vi "ContourPlot v3.6-IV.vi"() -> ()   [LabVIEW 2019]
uses:
  diff para.ctl
  graph para.ctl
panel:
  out "smoothed dIV buffer":dbl[][](array[numeric])
  in  "diff para":T1={"x0"=-1.0, "Ic0"=2.0, "h0"=1.0, "y0"=0.0}
  in  "Plot reference":bool caption="load data"
  out "smoothed dIV":dbl[][](array[numeric])
  out "smoothed data":dbl[][](array[numeric])
  in  "smooth n":i32=10
  out "IVdata":dbl[][](array[numeric])
  in  "load data":bool
  out "Status":string
  in  "stop":bool
  in  "Begin":i32=1000
  in  "length":i32=1000
  in  "Contact Resistance":dbl
  in  "Tab Control 2":enum32{"IV plots", "IV smoothed", "dV/dI"}(tab)
  out "IV Intensity":dbl[][](graph)
  out "IV":cluster{dbl[], "Intensity Graph":dbl[]}(graph)
  in  "Plot contour line":bool
  out "IV smoothed intensity":dbl[][](graph)
  out "Smooth IV":cluster{dbl[], "Intensity Graph":dbl[]}(graph)
  out "dVdI Intensity":dbl[][](graph)
  out "dV/dI":cluster{dbl[], "Intensity Graph":dbl[]}(graph)
  in  "book number":i32=414
  in  "file path (dialog if empty)":path=path "C:/Users/gyue/Box/Guang Yue uiuc research box folder/data/Contour plot"
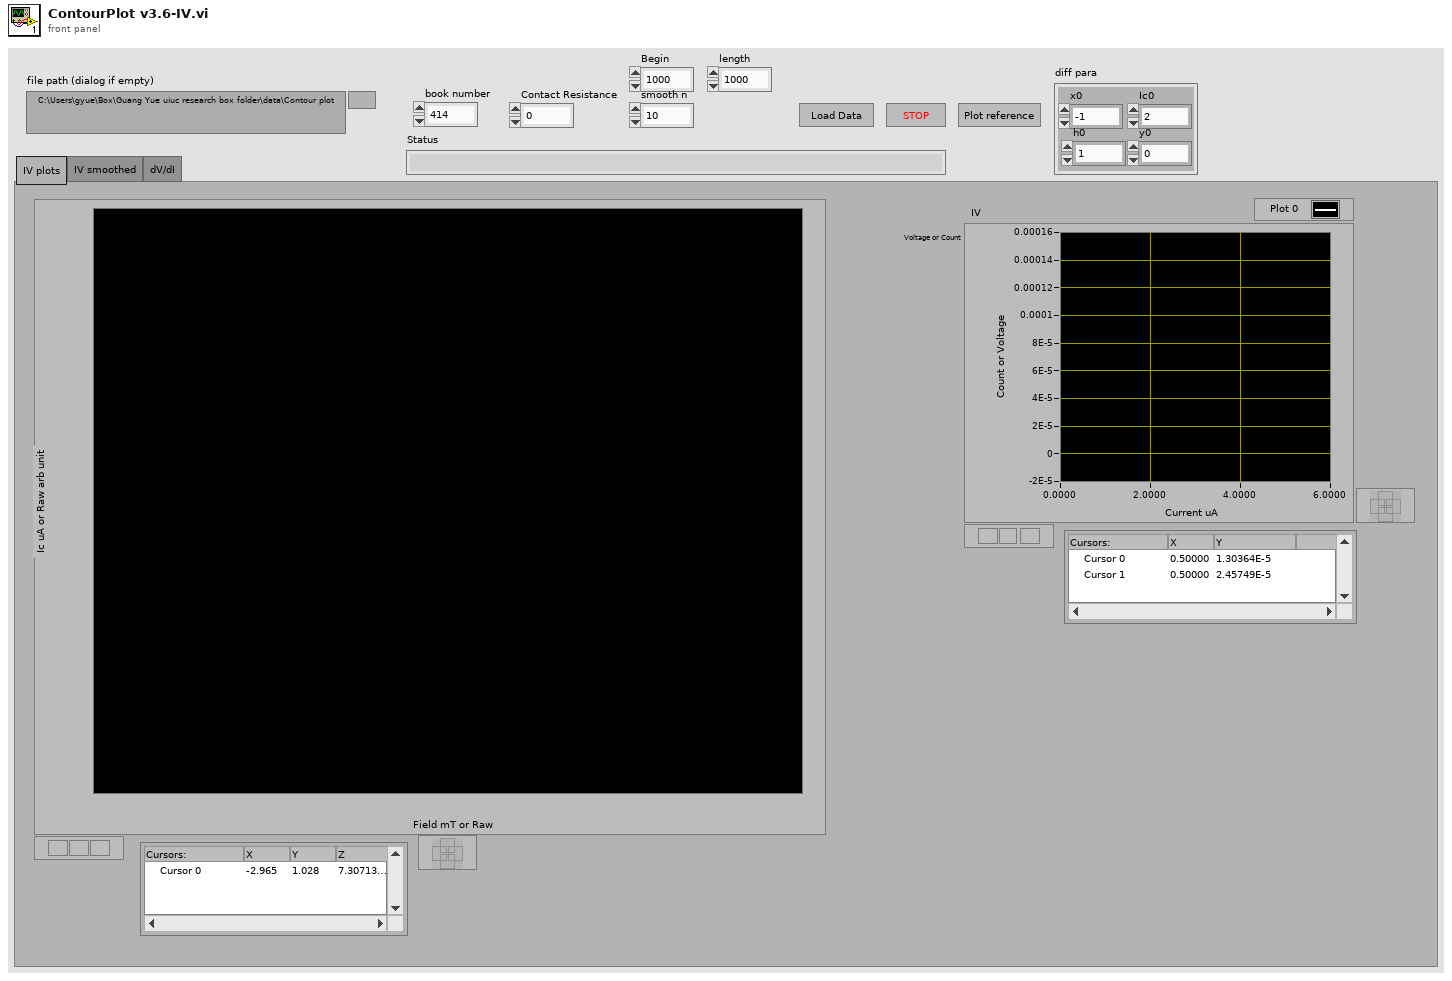
[diagram p1: front panel]
types:
  T1 = typedef "diff para.ctl" = cluster{"x0":dbl, "Ic0":dbl, "h0":dbl, "y0":dbl}
  T2 = typedef "graph para.ctl" = cluster{"x offset":dbl, "y offset":dbl, "x scale":dbl, "y scale":dbl}
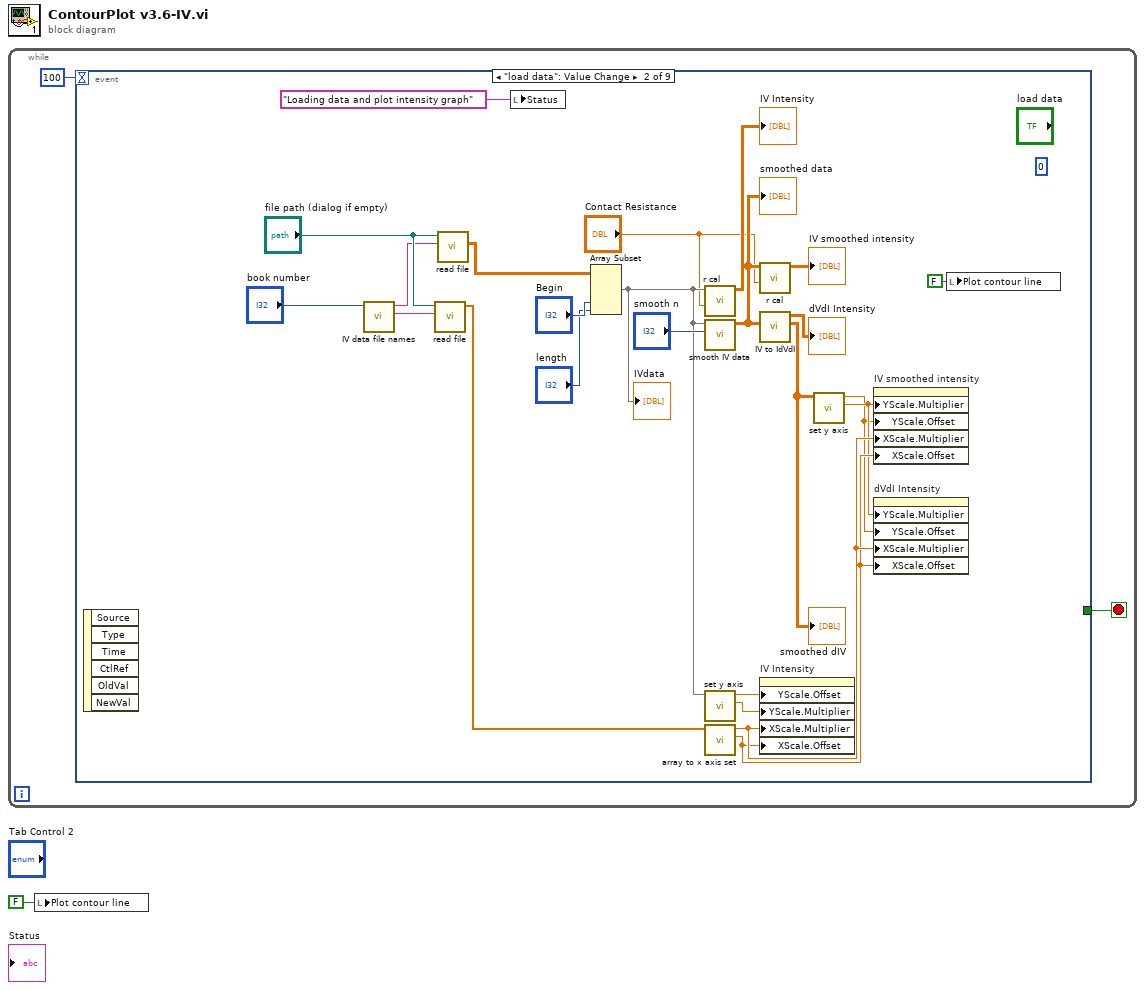
[diagram p0: block diagram]
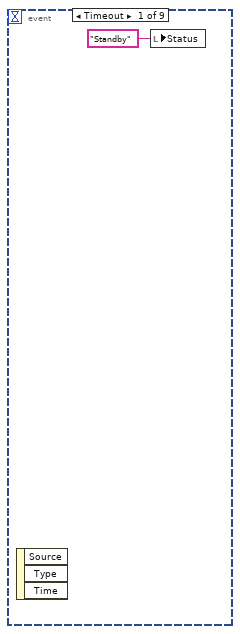
[diagram p2: hidden frame]
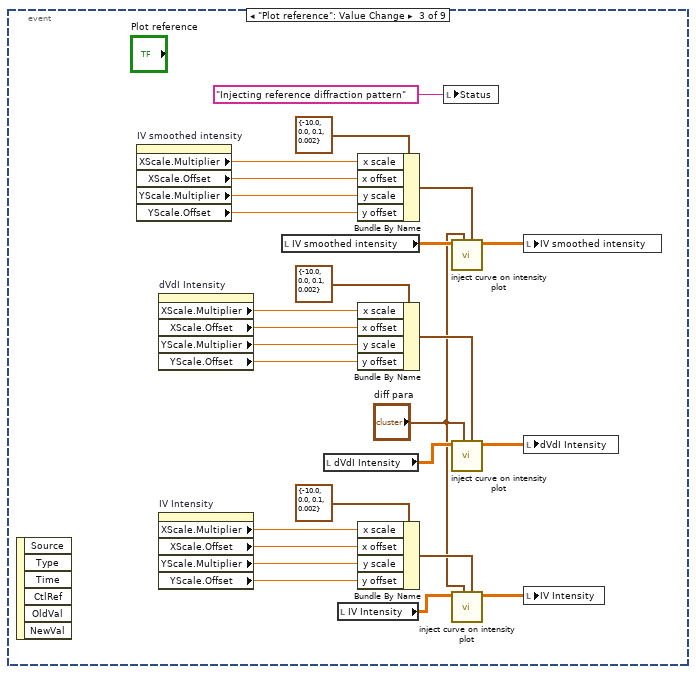
[diagram p3: hidden frame]
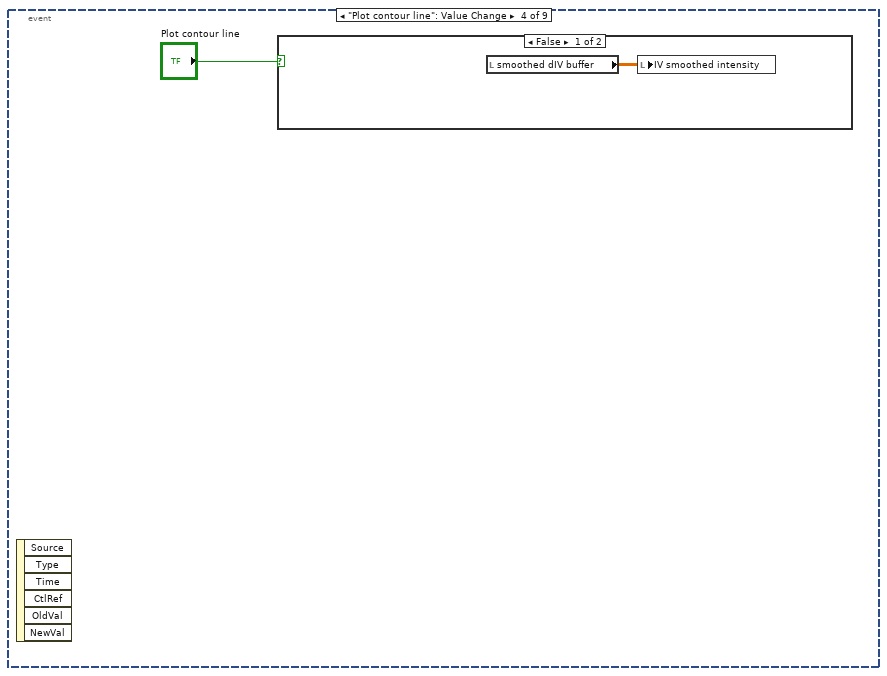
[diagram p4: hidden frame]
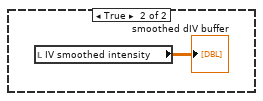
[diagram p5: hidden frame]
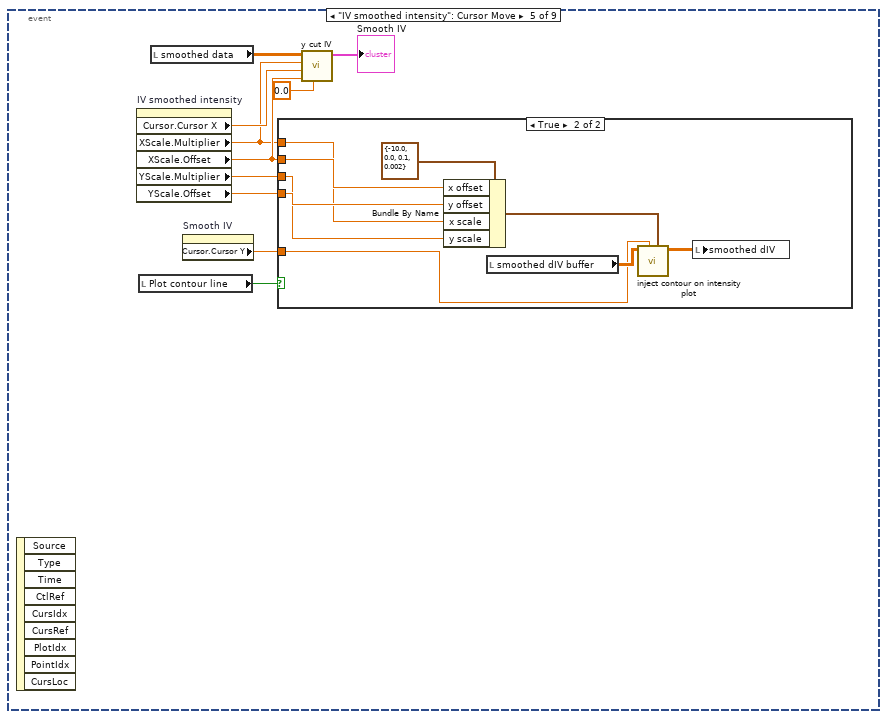
[diagram p6: hidden frame]
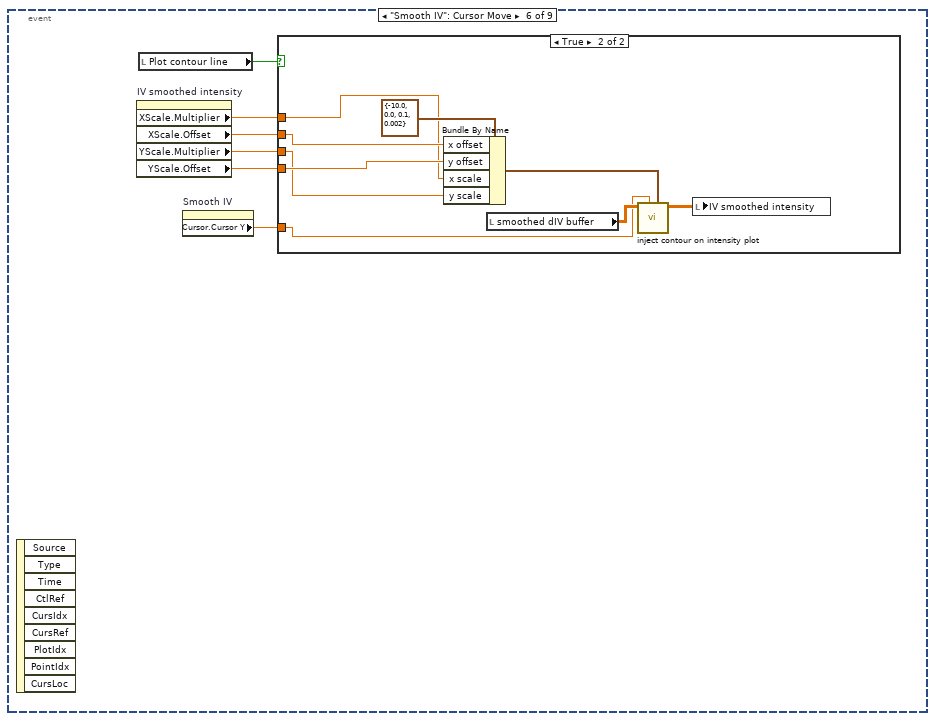
[diagram p8: hidden frame]
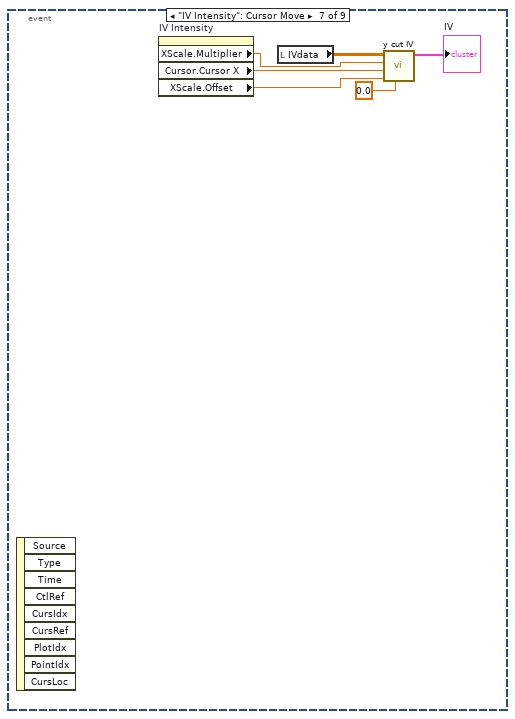
[diagram p10: hidden frame]
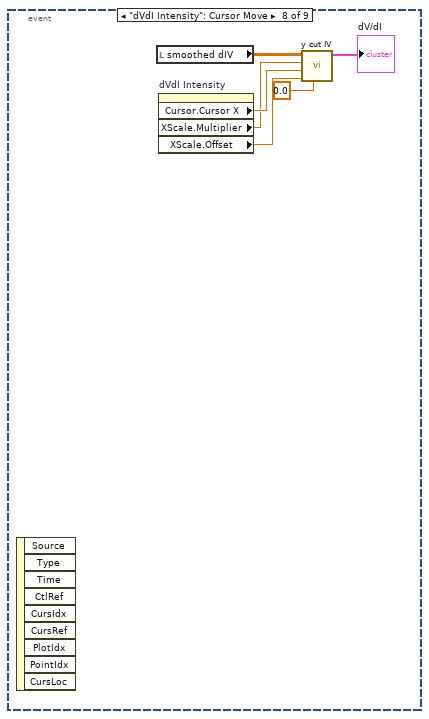
[diagram p11: hidden frame]
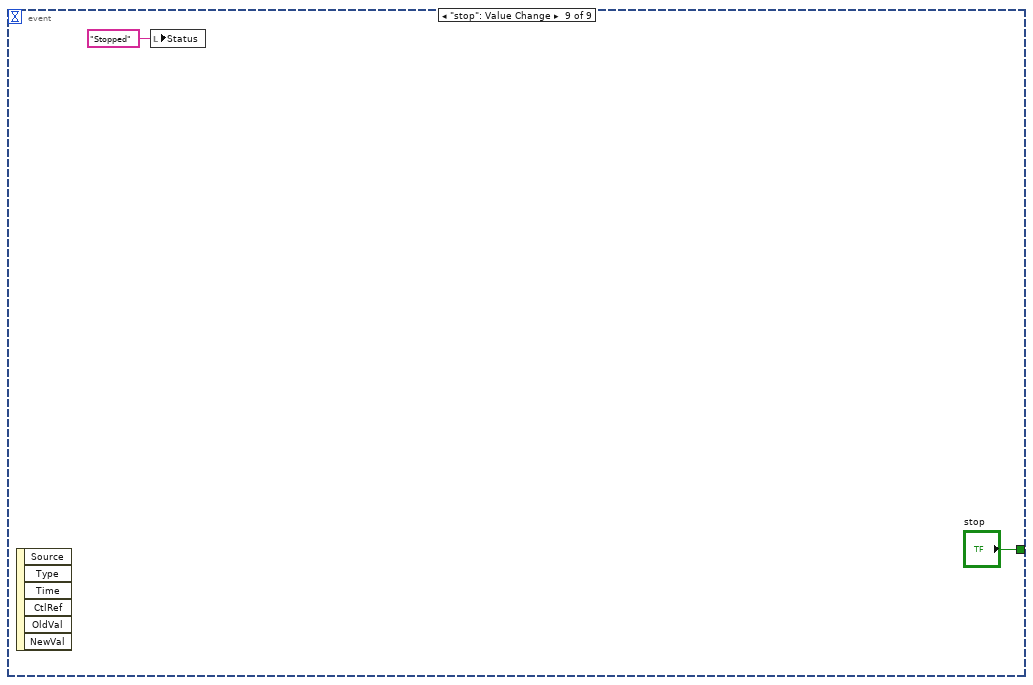
[diagram p12: hidden frame]
diagram:
  n1 = while {
    stop <- w2 stop-if-true
    n2 = event shown="[1] \"load data\": Value Change" {
      selector: _ -> [_ _ _ _ _ _ _ _ _]
      dyn-events: _ -> [_ _ _ _ _ _ _ _ _]
      timeout: 100 -> [_ _ _ _ _ _ _ _ _]
      tunnel: [_ _ _ _ _ _ _ _ "stop"] -> w2
      event Timeout {
        n3 = event-data() -> ()  [unwired: 1 in, 3 out]
        n4 = local write "Status"("Standby" ("Status")) -> ()
      }
      event "load data": Value Change {
        (unwired) 0 ("index (row)")
        n5 = event-data() -> ()  [unwired: 1 in, 6 out]
        n6 = call "IV data file names.vi"("book number"="book number") -> ("Field"=w27:string, "IV"=w25:string)  [unwired: 8 in, 1 out]
        n7 = call "read file.vi"("file name"=w27, "file path (dialog if empty)"="file path (dialog if empty)") -> ("1d Data"=w17:dbl[])  [unwired: 8 in, 1 out]
        n8 = call "read file.vi"("file name"=w25, "file path (dialog if empty)"="file path (dialog if empty)") -> ("2d data"=w18:dbl[][])  [unwired: 8 in, 1 out]
        n9 = local write "Status"("Loading data and plot intensity graph" ("Status")) -> ()
        n10 = Array Subset(array=w18, index (col)="Begin", length (col)="length") -> (w14:dbl[][])  [unwired: 2 in]
        "IVdata" <- w14
        n11 = call "r cal.vi"("Contact Resistance"="Contact Resistance", "Array in"=w14) -> ("Array out"=→"IV Intensity":dbl[][])  [unwired: 9 in]
        n12 = call "smooth IV data.vi"("smooth n"="smooth n", "Array in"=w14) -> ("Array out"=w13:dbl[][])  [unwired: 9 in]
        "smoothed data" <- w13
        n13 = call "set y axis.vi"("Array"=w14) -> ("y multi"=w24:dbl, "y offset"=w23:dbl)  [unwired: 9 in]
        n14 = call "array to x axis set.vi"("1d Data"=w17) -> ("offset"=w9:dbl, "multiplier"=w10:dbl)  [unwired: 9 in]
        n15 = call "r cal.vi"("Contact Resistance"="Contact Resistance", "Array in"=w13) -> ("Array out"=→"IV smoothed intensity":dbl[][])  [unwired: 9 in]
        n16 = call "IV to IdVdI.vi"("Array in"=w13) -> ("Array"=w8:dbl[][], "Array 2"=→"dVdI Intensity":dbl[][])  [unwired: 9 in]
        "smoothed dIV" <- w8
        n17 = property on="IV Intensity" class="IntGraph (strict)"("YScale.Offset"=w23, "YScale.Multiplier"=w24, "XScale.Multiplier"=w10, "XScale.Offset"=w9) -> ()  [unwired: 2 in, 2 out]
        n18 = call "set y axis.vi"("Array"=w8) -> ("y multi"=w7:dbl, "y offset"=w6:dbl)  [unwired: 9 in]
        n19 = property on="IV smoothed intensity" class="IntGraph (strict)"("YScale.Multiplier"=w7, "YScale.Offset"=w6, "XScale.Multiplier"=w10, "XScale.Offset"=w9) -> ()  [unwired: 2 in, 2 out]
        n20 = property on="dVdI Intensity" class="IntGraph (strict)"("YScale.Multiplier"=w7, "YScale.Offset"=w6, "XScale.Multiplier"=w10, "XScale.Offset"=w9) -> ()  [unwired: 2 in, 2 out]
        n21 = local write "Plot contour line"(FALSE ("Plot contour line")) -> ()
      }
      event "Plot reference": Value Change {
        n22 = event-data() -> ()  [unwired: 1 in, 6 out]
        n23 = property on="IV smoothed intensity" class="IntGraph (strict)"() -> ("XScale.Multiplier"=w40:dbl, "XScale.Offset"=w39:dbl, "YScale.Multiplier"=w38:dbl, "YScale.Offset"=w37:dbl)  [unwired: 2 in, 2 out]
        n24 = property on="dVdI Intensity" class="IntGraph (strict)"() -> ("XScale.Multiplier"=w34:dbl, "XScale.Offset"=w33:dbl, "YScale.Multiplier"=w32:dbl, "YScale.Offset"=w31:dbl)  [unwired: 2 in, 2 out]
        n25 = property on="IV Intensity" class="IntGraph (strict)"() -> ("XScale.Multiplier"=w52:dbl, "XScale.Offset"=w51:dbl, "YScale.Multiplier"=w50:dbl, "YScale.Offset"=w49:dbl)  [unwired: 2 in, 2 out]
        n26 = local read "IV smoothed intensity"() -> (w41:dbl[][])
        n27 = local read "dVdI Intensity"() -> (w35:dbl[][])
        n28 = local read "IV Intensity"() -> (w54:dbl[][])
        n29 = Bundle By Name(cluster=T2 {"x offset"=-10.0, "y offset"=0.0, "x scale"=0.1, "y scale"=0.002} ("graph para"), "x scale"=w40, "x offset"=w39, "y scale"=w38, "y offset"=w37) -> (w44:T2)
        n30 = Bundle By Name(cluster=T2 {"x offset"=-10.0, "y offset"=0.0, "x scale"=0.1, "y scale"=0.002} ("graph para"), "x scale"=w34, "x offset"=w33, "y scale"=w32, "y offset"=w31) -> (w42:T2)
        n31 = Bundle By Name(cluster=T2 {"x offset"=-10.0, "y offset"=0.0, "x scale"=0.1, "y scale"=0.002} ("graph para"), "x scale"=w52, "x offset"=w51, "y scale"=w50, "y offset"=w49) -> (w48:T2)
        n32 = local write "Status"("Injecting reference diffraction pattern" ("Status")) -> ()
        n33 = call "inject curve on intensity plot.vi"("graph para"=w44, "diff para"="diff para", "IV Intensity"=w41) -> ("IV Intensity 2"=w36:dbl[][])  [unwired: 8 in]
        n34 = call "inject curve on intensity plot.vi"("graph para"=w42, "diff para"="diff para", "IV Intensity"=w35) -> ("IV Intensity 2"=w29:dbl[][])  [unwired: 8 in]
        n35 = call "inject curve on intensity plot.vi"("graph para"=w48, "diff para"="diff para", "IV Intensity"=w54) -> ("IV Intensity 2"=w47:dbl[][])  [unwired: 8 in]
        n36 = local write "IV smoothed intensity"(w36) -> ()
        n37 = local write "dVdI Intensity"(w29) -> ()
        n38 = local write "IV Intensity"(w47) -> ()
      }
      event "Plot contour line": Value Change {
        n39 = event-data() -> ()  [unwired: 1 in, 6 out]
        n40 = case shown="False" "Plot contour line" {
          frame False {
            n41 = local read "smoothed dIV buffer"() -> (w56:dbl[][])
            n42 = local write "IV smoothed intensity"(w56) -> ()
          }
          frame True {
            n43 = local read "IV smoothed intensity"() -> (→"smoothed dIV buffer":dbl[][])
          }
        }
      }
      event "IV smoothed intensity": Cursor Move {
        n44 = event-data() -> ()  [unwired: 1 in, 9 out]
        n45 = property on="IV smoothed intensity" class="IntGraph (strict)"() -> ("Cursor.Cursor X"=w64:dbl, "XScale.Multiplier"=w60:dbl, "XScale.Offset"=w62:dbl, "YScale.Multiplier"=w59:dbl, "YScale.Offset"=w61:dbl)  [unwired: 2 in, 2 out]
        n46 = local read "Plot contour line"() -> (w63:bool)
        n47 = local read "smoothed data"() -> (w67:dbl[][])
        n48 = property on="Smooth IV" class="XYGraph (strict)"() -> ("Cursor.Cursor Y"=w58:dbl)  [unwired: 2 in, 2 out]
        n49 = case shown="True" w63 {
          tunnel: w58 -> [_ w74]
          tunnel: w62 -> [_ w72]
          tunnel: w61 -> [_ w71]
          tunnel: w60 -> [_ w70]
          tunnel: w59 -> [_ w69]
          frame False {
          }
          frame True {
            n50 = Bundle By Name(cluster=T2 {"x offset"=-10.0, "y offset"=0.0, "x scale"=0.1, "y scale"=0.002} ("graph para"), "x offset"=w72, "y offset"=w71, "x scale"=w70, "y scale"=w69) -> (w68:T2)
            n51 = local read "smoothed dIV buffer"() -> (w76:dbl[][])
            n52 = call "inject contour on intensity plot.vi"("graph para"=w68, "Threshold"=w74, "IV Intensity"=w76) -> ("IV Intensity output"=w75:dbl[][])  [unwired: 6 in, 2 out]
            n53 = local write "smoothed dIV"(w75) -> ()
          }
        }
        n54 = call "y cut IV.vi"("Contact Resistance"=0.0, "x offset"=w62, "x pos"=w64, "scale"=w60, "Data"=w67) -> ("IV"=→"Smooth IV":cluster{"Data":dbl[], dbl[]})  [unwired: 6 in]
      }
      event "Smooth IV": Cursor Move {
        n55 = event-data() -> ()  [unwired: 1 in, 9 out]
        n56 = property on="IV smoothed intensity" class="IntGraph (strict)"() -> ("XScale.Multiplier"=w79:dbl, "XScale.Offset"=w81:dbl, "YScale.Multiplier"=w78:dbl, "YScale.Offset"=w80:dbl)  [unwired: 2 in, 2 out]
        n57 = local read "Plot contour line"() -> (w82:bool)
        n58 = property on="Smooth IV" class="XYGraph (strict)"() -> ("Cursor.Cursor Y"=w77:dbl)  [unwired: 2 in, 2 out]
        n59 = case shown="True" w82 {
          tunnel: w77 -> [_ w89]
          tunnel: w81 -> [_ w87]
          tunnel: w80 -> [_ w86]
          tunnel: w79 -> [_ w85]
          tunnel: w78 -> [_ w84]
          frame False {
          }
          frame True {
            n60 = Bundle By Name(cluster=T2 {"x offset"=-10.0, "y offset"=0.0, "x scale"=0.1, "y scale"=0.002} ("graph para"), "x offset"=w87, "y offset"=w86, "x scale"=w85, "y scale"=w84) -> (w83:T2)
            n61 = local read "smoothed dIV buffer"() -> (w91:dbl[][])
            n62 = call "inject contour on intensity plot.vi"("graph para"=w83, "Threshold"=w89, "IV Intensity"=w91) -> ("IV Intensity output"=w90:dbl[][])  [unwired: 6 in, 2 out]
            n63 = local write "IV smoothed intensity"(w90) -> ()
          }
        }
      }
      event "IV Intensity": Cursor Move {
        n64 = event-data() -> ()  [unwired: 1 in, 9 out]
        n65 = property on="IV Intensity" class="IntGraph (strict)"() -> ("XScale.Multiplier"=w94:dbl, "Cursor.Cursor X"=w95:dbl, "XScale.Offset"=w96:dbl)  [unwired: 2 in, 2 out]
        n66 = local read "IVdata"() -> (w93:dbl[][])
        n67 = call "y cut IV.vi"("Contact Resistance"=0.0, "x offset"=w96, "x pos"=w95, "scale"=w94, "Data"=w93) -> ("IV"=→"IV":cluster{"Data":dbl[], dbl[]})  [unwired: 6 in]
      }
      event "dVdI Intensity": Cursor Move {
        n68 = event-data() -> ()  [unwired: 1 in, 9 out]
        n69 = local read "smoothed dIV"() -> (w103:dbl[][])
        n70 = property on="dVdI Intensity" class="IntGraph (strict)"() -> ("Cursor.Cursor X"=w101:dbl, "XScale.Multiplier"=w100:dbl, "XScale.Offset"=w99:dbl)  [unwired: 2 in, 2 out]
        n71 = call "y cut IV.vi"("Contact Resistance"=0.0, "x offset"=w99, "x pos"=w101, "scale"=w100, "Data"=w103) -> ("IV"=→"dV/dI":cluster{"Data":dbl[], dbl[]})  [unwired: 6 in]
      }
      event "stop": Value Change {
        n72 = event-data() -> ()  [unwired: 1 in, 6 out]
        n73 = local write "Status"("Stopped" ("Status")) -> ()
      }
    }
  }
  n74 = local write "Plot contour line"(FALSE ("Plot contour line")) -> ()
